vi "K_S30_VISA F69.vi"(4 "error in":errorcluster, 7 "Address":u8=250) -> (0 "error out":errorcluster, 3 "Serial Nr.":u32)   [LabVIEW 2012]
panel:
  # "Function 69: Read Serial Nr\nV1.0, b.v."
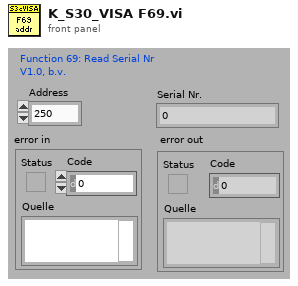
[diagram p1: front panel]
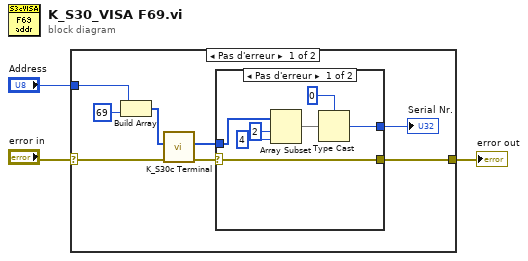
[diagram p0: block diagram]
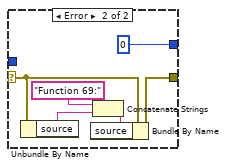
[diagram p2: hidden frame]
diagram:
  n1 = case shown="Pas d'erreur" "error in" {
    selector: "error in" -> [w8 w25]
    tunnel: "Address" -> [w11 _]
    tunnel: [w6 w25] -> w1
    frame No Error {
      n2 = Build Array(w11, u8 69 ("Element")) -> (w9:u8[])
      n3 = call "K_S30c Terminal.vi"("error in"=w8, "request"=w9) -> ("error out"=w7:errorcluster, "response"=w5:u8[])  [unwired: 4 in]
      n4 = case shown="Pas d'erreur" w7 {
        selector: w7 -> [w18 w24]
        tunnel: [w18 w22] -> w6
        tunnel: w5 -> [w17 _]
        tunnel: [w13 u32 0] -> w4
        frame No Error {
          n5 = Array Subset(array=w17, index=2 ("Index"), length=4 ("Länge")) -> (w12:u8[])
          n6 = Type Cast(type=u32 0, x=w12) -> (*(type *) &x=w13:u32)
        }
        frame Error {
          n7 = Unbundle By Name(w24) -> ("source"=w20:string)
          n8 = Concatenate Strings("Function 69:" ("String"), w20) -> (w23:string)
          n9 = Bundle By Name(cluster=w24, "source"=w23) -> (w22:errorcluster)
        }
      }
      "Serial Nr." <- w4
    }
    frame Error {
    }
  }
  "error out" <- w1
